vi "ADIS16470 Globals.vi"() -> ()   [LabVIEW 2019]
panel:
  out "TempDegC":dbl
  out "DiagStat":u16
  out "Offset Bias":u16[](array[numeric])
  out "Loop State":i32
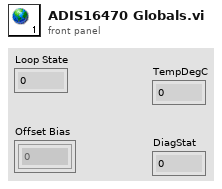
[diagram p1: front panel]
diagram:
